vi "Field.vi"(4 "channel 2":T8, 6 "Draw Targets?":T7, 7 "AutoScale":bool=TRUE, 8 "channel for IA State":T9, 10 "Scale mm/pixel":dbl=1.0 format="%#_13g", 11 "channel":T1) -> (2 "Scale Out":dbl, 3 "2D Picture":picture, 5 "AutoScale Out":bool=TRUE)   [LabVIEW 2017]
uses:
  <extravilib>/ChannelInstances/Lossy Stream-t'AI Input.ctl'/)Channel.ctl
  Core/AI Input.ctl
  Core/AI Robot.ctl
  Intel/Functions Enum.ctl
  Intel/AttackerStates.ctl
  Path Planning/RRT/PathDests.ctl
  Path Planning/RRT/PathDest.ctl
  Core/AI Ball.ctl
  Core/Field Size.ctl
  Core/AI Judge.ctl
  Intel/Command Enum.ctl
  Util/Events/Events.ctl
  <extravilib>/ChannelInstances/Lossy Stream-a[.](i32)/)Channel.ctl
  DrawTargets.ctl
  SSL/SSL Field State.ctl
  SSL Detection Frame.ctl
  SSL Detection Robot.ctl
  <vilib>/Analysis/Matrix/Datatypes/RealMatrix.ctl
  SSL Detection Ball.ctl
  <extravilib>/ChannelInstances/Lossy Stream-t'VSS Field State.ctl'/)Channel.ctl
  SSL/VSS Field State.ctl
  <vilib>/Utility/miscctls.llb/LVBoundsTypeDef.ctl
  <extravilib>/ChannelInstances/Lossy Stream-t'VSS Field State.ctl'/Read With Abort.vi
  <extravilib>/ChannelInstances/Lossy Stream-a[.](i32)/Read With Abort.vi
  <extravilib>/ChannelInstances/Lossy Stream-t'AI Input.ctl'/Read With Abort.vi
  <extravilib>/ChannelInstances/Lossy Stream-t'VSS Field State.ctl'/EndpointRead.vi
  <extravilib>/ChannelInstances/Lossy Stream-a[.](i32)/EndpointRead.vi
  <extravilib>/ChannelInstances/Lossy Stream-t'AI Input.ctl'/EndpointRead.vi
  <extravilib>/ChannelInstances/Lossy Stream-t'AI Input.ctl'/)Channel.vi
  <resource>/ChannelSupport/_ChannelSupport/WaitIfNeeded.vi
  <extravilib>/ChannelInstances/Lossy Stream-a[.](i32)/)Channel.vi
  <extravilib>/ChannelInstances/Lossy Stream-t'VSS Field State.ctl'/)Channel.vi
  <extravilib>/ChannelInstances/Lossy Stream-t'AI Input.ctl'.lvlib
  <extravilib>/ChannelInstances/Lossy Stream-a[.](i32).lvlib
  <extravilib>/ChannelInstances/Lossy Stream-t'VSS Field State.ctl'.lvlib
  <vilib>/Analysis/Matrix/NI_Matrix.lvlib
panel:
  in  "element":T2 {"Detection Frame Out"."robots_blue"."height" format="%+4.3f"; "Detection Frame Out"."robots_blue"."pixel_y" format="%+4.3f"; "Detection Frame Out"."robots_blue"."pixel_x" format="%+4.3f"; "Detection Frame Out"."robots_blue"."orientation" format="%+4.3f"; "Detection Frame Out"."robots_blue"."y" format="%+4.3f"; "Detection Frame Out"."robots_blue"."confidence" format="%4.3f"; "Detection Frame Out"."robots_blue"."x" format="%+4.3f"; "Detection Frame Out"."robots_yellow"."height" format="%+4.3f"; "Detection Frame Out"."robots_yellow"."pixel_y" format="%+4.3f"; "Detection Frame Out"."robots_yellow"."pixel_x" format="%+4.3f"; "Detection Frame Out"."robots_yellow"."orientation" format="%+4.3f"; "Detection Frame Out"."robots_yellow"."y" format="%+4.3f"; "Detection Frame Out"."robots_yellow"."confidence" format="%4.3f"; "Detection Frame Out"."robots_yellow"."x" format="%+4.3f"}
  in  "Draw Number":bool=TRUE
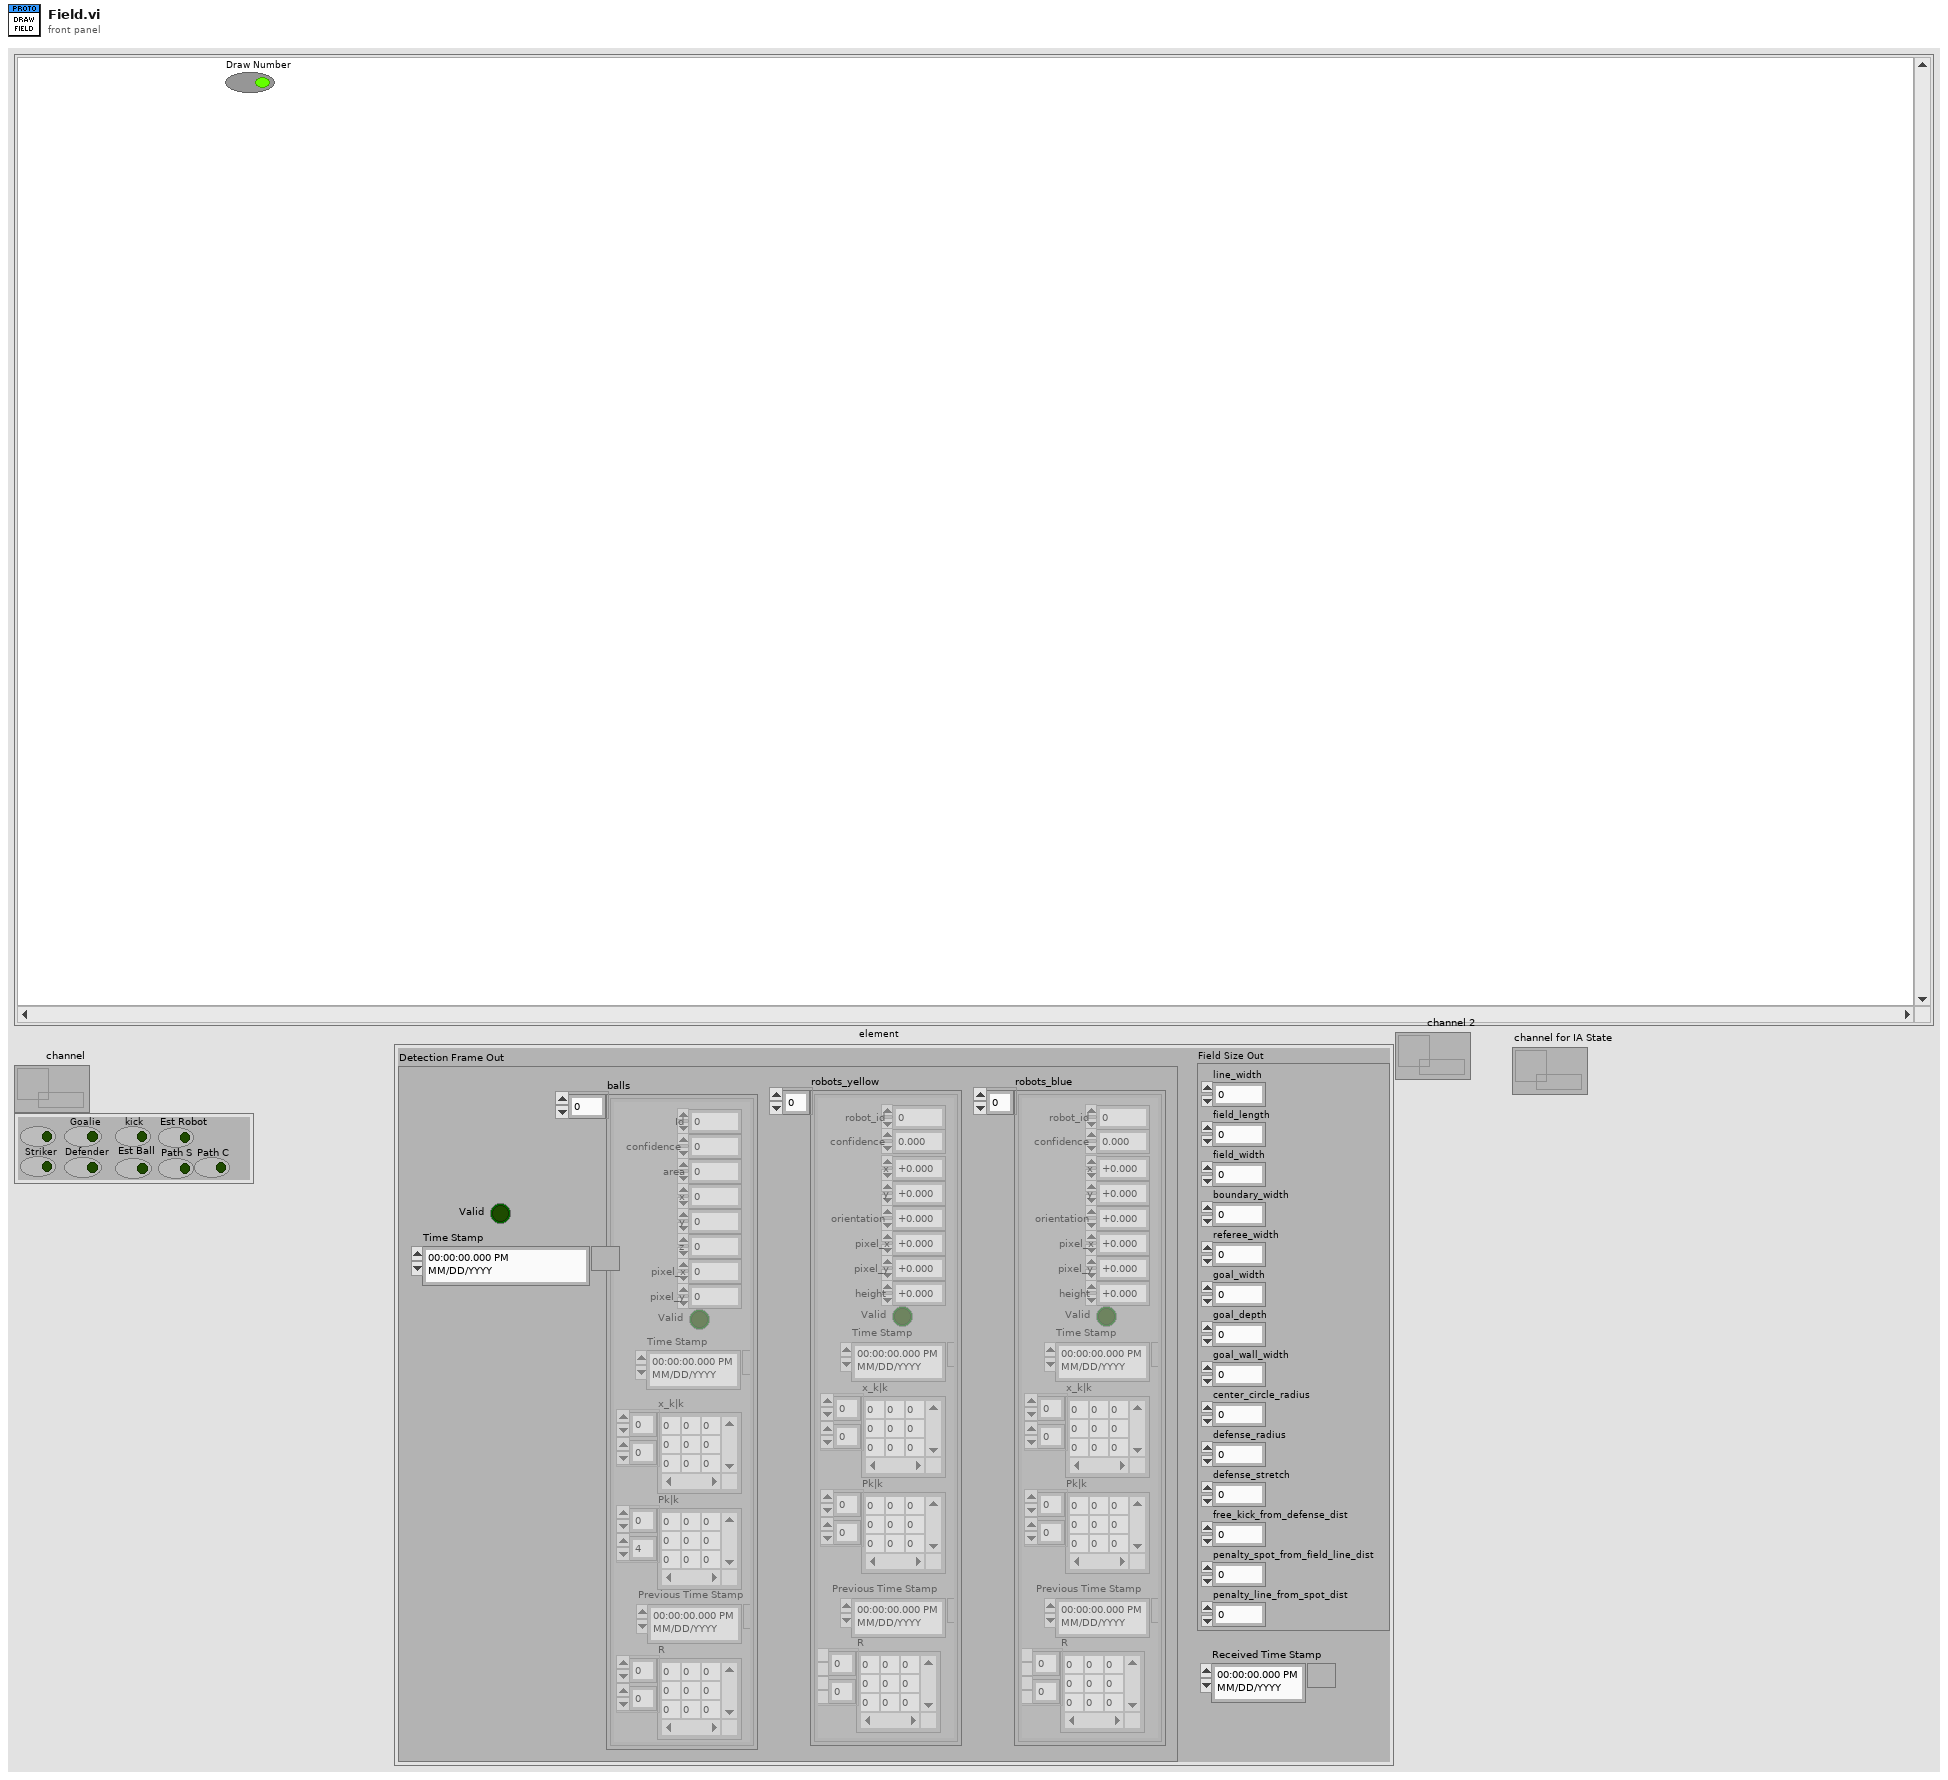
[diagram p1: front panel]
types:
  T1 = typedef "Lossy Stream-t'VSS Field State.ctl'.lvlib/)Channel.ctl" = refnum<queue>
  T2 = typedef "SSL Field State.ctl" = cluster{"Detection Frame Out":T3, "Field Size Out":cluster{"line_width":u32, "field_length":u32, "field_width":u32, "boundary_width":u32, "referee_width":u32, "goal_width":u32, "goal_depth":u32, "goal_wall_width":u32, "center_circle_radius":u32, "defense_radius":u32, "defense_stretch":u32, "free_kick_from_defense_dist":u32, "penalty_spot_from_field_line_dist":u32, "penalty_line_from_spot_dist":u32}, "Received Time Stamp":timestamp}
  T3 = typedef "SSL Detection Frame.ctl" = cluster{"robots_yellow":T4[], "robots_blue":T4[], "balls":T6[], "Valid":bool, "Time Stamp":timestamp}
  T4 = typedef "SSL Detection Robot.ctl" = cluster{"x":sgl, "robot_id":u32, "confidence":sgl, "y":sgl, "orientation":sgl, "pixel_x":sgl, "pixel_y":sgl, "height":sgl, "Valid":bool, "Time Stamp":timestamp, "x_k|k":T5, "Pk|k":T5, "Previous Time Stamp":timestamp, "R":T5}
  T5 = typedef "NI_Matrix.lvlib/RealMatrix.ctl" = dbl[][]
  T6 = typedef "SSL Detection Ball.ctl" = cluster{"x":sgl, "area":u32, "confidence":sgl, "y":sgl, "z":sgl, "pixel_x":sgl, "pixel_y":sgl, "Valid":bool, "Time Stamp":timestamp, "x_k|k":T5, "Pk|k":T5, "Id":u32, "Previous Time Stamp":timestamp, "R":T5}
  T7 = typedef "DrawTargets.ctl" = cluster{"Attacker":bool, "Striker":bool, "Goalie":bool, "Defender":bool, "kick":bool, "Est Ball":bool, "Est Robot":bool, "Path S":bool, "Path C":bool}
  T8 = typedef "Lossy Stream-a[.](i32).lvlib/)Channel.ctl" = refnum<queue>
  T9 = typedef "Lossy Stream-t'AI Input.ctl'.lvlib/)Channel.ctl" = refnum<queue>
  T10 = typedef "LVBoundsTypeDef.ctl" = cluster{"Width":u32, "Height":u32}
  T11 = typedef "VSS Field State.ctl" = cluster{"Detection Frame Out":T3, "Received Time Stamp":timestamp, "Field Size in":cluster{"field_length":u32, "field_width":u32, "goal_width":u32, "goal_depth":u32, "center_circle_radius":u32, "defense_width":u32, "defense_depth":u32, "free_kick_from_defense_dist":u32, "penalty_spot_from_field_line_dist":u32, "penalty_line_from_spot_dist":u32, "half_moon_depth":u32, "half_moon_width":u32}}
  T12 = typedef "AI Input.ctl" = cluster{"our_robots":T13[], "enemy_robots":T13[], "balls":T18[], "geometry":T19, "IA Judge":T20, "Received Timestamp":timestamp, "Events":T22}
  T13 = typedef "AI Robot.ctl" = cluster{"id":u32, "function":T14, "x":dbl, "y":dbl, "orientation":dbl, "v_tangent":dbl, "v_normal":dbl, "v_ang":dbl, "kick_x":dbl, "kick_z":dbl, "dribble":bool, "Timestamp":timestamp, "estimatives":cluster{"est_v_tangent":dbl, "est_v_normal":dbl, "est_vx":dbl, "est_vy":dbl, "Pos Robot Est":dbl[]}, "dest_x_kick":dbl, "dest_y_kick":dbl, "Gap Coord":dbl[], "States":T15, "Path ":dbl[][], "Path  Smooth":dbl[][], "Dest":T16}
  T14 = typedef "Functions Enum.ctl" = enum16{"Attacker", "Goalie", "Defender", "Striker", "Goto 0", "Dummy", "Kicker", "ZigZag"}
  T15 = typedef "AttackerStates.ctl" = enum16{"Pass", "GoToTangent", "BallGetting", "GoToKick", ""}
  T16 = typedef "PathDests.ctl" = T17[]
  T17 = typedef "PathDest.ctl" = cluster{"dest_x":dbl, "dest_y":dbl, "dest_orientation":dbl, "dest_vel":dbl}
  T18 = typedef "AI Ball.ctl" = cluster{"x":dbl, "y":dbl, "timestamp":timestamp, "Vel_x":dbl, "Vel_y":dbl, "Pos Bola Est":dbl[]}
  T19 = typedef "Field Size.ctl" = cluster{"line_width":u32, "field_length":u32, "field_width":u32, "boundary_width":u32, "referee_width":u32, "goal_width":u32, "goal_depth":u32, "goal_wall_width":u32, "center_circle_radius":u32, "defense_radius":u32, "defense_stretch":u32, "free_kick_from_defense_dist":u32, "penalty_spot_from_field_line_dist":u32, "penalty_line_from_spot_dist":u32}
  T20 = typedef "AI Judge.ctl" = cluster{"stage":string, "command":string, "our_goalie_id":dbl, "enemy_goalie_id":dbl, "command enum":T21, "Time":enum16{"Azul", "Amarelo"}}
  T21 = typedef "Command Enum.ctl" = enum16{"Halt", "Stop", "Force Start", "PKA Normal Start", "Prepare Kickoff Ally", "PKE Normal Start", "Prepare Kickoff Enemy", "Prepare Penalty Ally", "PPA Normal Start", "Prepare Penalty Enemy", "PPE Normal Start", "Direct Free Enemy", "Direct Free Ally", "Indirect Free Enemy", "Indirect Free Ally", "Timeout Enemy", "Timeout Ally", "Goal Enemy", "Goal Ally", "Ball Placement Enemy", "Ball Placement Ally", "Normal Half Time", "Extra Time Break", "Extra Half Time", "None", "Post Game"}
  T22 = typedef "Events.ctl" = cluster{"Touch":bool, "Ball out":bool, "id touch":dbl, "Ball out of \nVision":bool, "Ball inside \nGoalie area":bool, "Robot not responding":bool, "Robots responding status":dbl[], "Enemy Ball \nPossession":bool, "Pass State":bool, "id end of pass":dbl, "Kick":bool, "Id ini Possession":dbl, "Ball Possesion":bool, "Id Possesion":dbl}
  T23 = cluster{"field_length":u32, "field_width":u32, "goal_width":u32, "goal_depth":u32, "center_circle_radius":u32, "defense_width":u32, "defense_depth":u32, "free_kick_from_defense_dist":u32, "penalty_spot_from_field_line_dist":u32, "penalty_line_from_spot_dist":u32, "half_moon_depth":u32, "half_moon_width":u32}
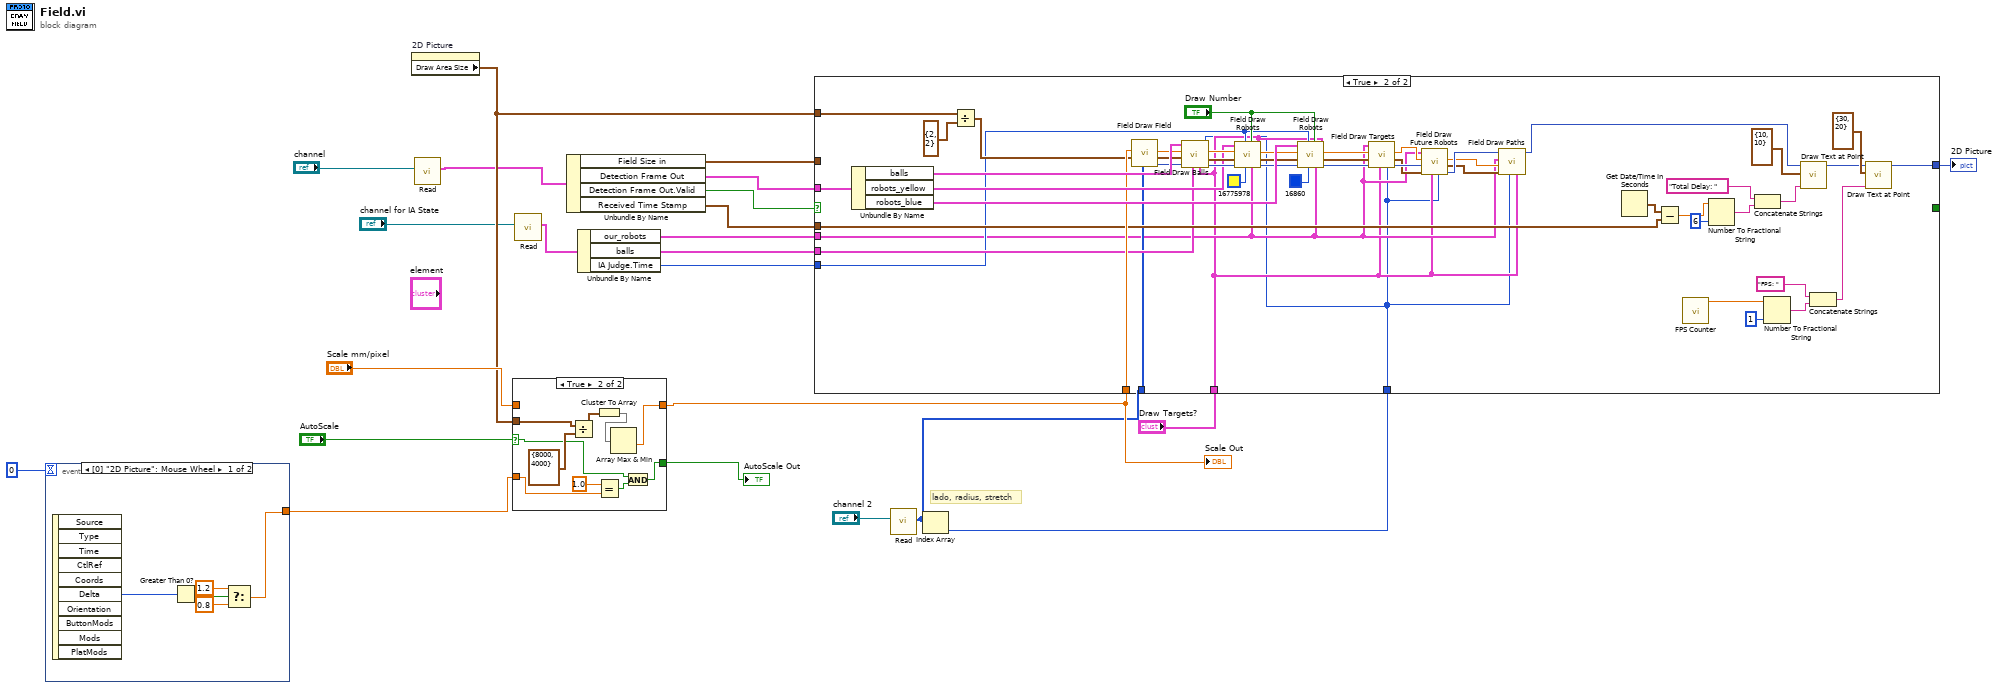
[diagram p0: block diagram]
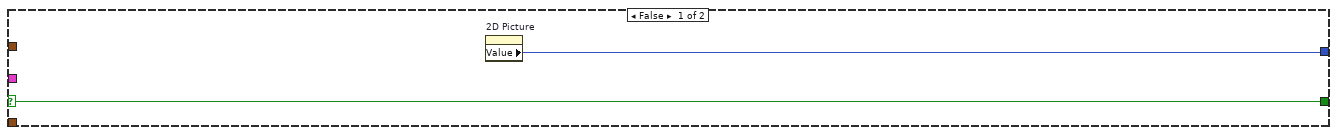
[diagram p2: hidden frame]
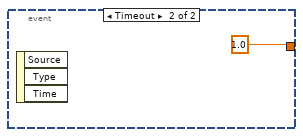
[diagram p3: hidden frame]
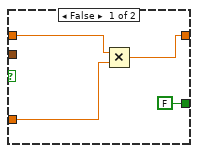
[diagram p4: hidden frame]
diagram:
  # "lado, radius, stretch"
  n1 = event shown="[0] \"2D Picture\": Mouse Wheel" {
    selector: _ -> [_ _]
    dyn-events: _ -> [_ _]
    timeout: 0 -> [_ _]
    tunnel: [w24 1.0] -> w21
    event "2D Picture": Mouse Wheel {
      n2 = event-data() -> ("Delta"=w28:i32)  [unwired: 1 in, 9 out]
      n3 = Greater Than 0?(x=w28) -> (x > 0?=w27:bool)
      n4 = Select(t=1.2, s=w27, f=0.8) -> (s? t:f=w24:dbl)
    }
    event Timeout {
      n5 = event-data() -> ()  [unwired: 1 in, 3 out]
    }
  }
  n6 = property on="2D Picture" class="Pict"() -> ("Draw Area Size"=w20:T10)  [unwired: 2 in, 2 out]
  n7 = call <extravilib>:"Read.vi"("channel"="channel") -> ("element"=w1:T11)  [unwired: 5 in, 5 out]
  n8 = case shown="True" "AutoScale" {
    selector: "AutoScale" -> [_ w35]
    tunnel: "Scale mm/pixel" -> [w33 _]
    tunnel: [w32 w39] -> w15
    tunnel: w20 -> [_ w43]
    tunnel: w21 -> [w31 w38]
    tunnel: [FALSE w36] -> w18
    frame False {
      n9 = Multiply(x=w33, y=w31) -> (x*y=w32:dbl)
    }
    frame True {
      n10 = Divide(x=w43, y=T10 {"Width"=8000, "Height"=4000}) -> (x/y=w41:cluster{"Width":dbl, "Height":dbl})
      n11 = Cluster To Array(cluster=w41) -> (array=w40:dbl[])
      n12 = Equal?(x=1.0, y=w38) -> (x = y?=w34:bool)
      n13 = Array Max & Min(array=w40) -> (min value=w39:dbl)  [unwired: 3 out]
      n14 = And(x=w35, y=w34) -> (x .and. y?=w36:bool)
    }
  }
  "Scale Out" <- w15
  "AutoScale Out" <- w18
  n15 = call <extravilib>:"Read.vi"("channel"="channel for IA State") -> ("element"=w12:T12)  [unwired: 5 in, 5 out]
  n16 = Unbundle By Name(w1) -> ("Field Size in"=w16:T23, "Detection Frame Out"=w17:T3, "Detection Frame Out.Valid"=w14:bool, "Received Time Stamp"=w13:timestamp)
  n17 = Unbundle By Name(w12) -> ("our_robots"=w3:T13[], "balls"=w7:T18[], "IA Judge.Time"=w4:enum16{"Azul", "Amarelo"})
  n18 = call <extravilib>:"Read.vi"("channel"="channel 2") -> ("element"=w5:i32[])  [unwired: 5 in, 5 out]
  n19 = Index Array(array=w5) -> (element=w10:i32)  [unwired: 1 in]
  n20 = case shown="True" w14 {
    selector: w14 -> [w45 _]
    tunnel: w20 -> [_ w96]
    tunnel: [w44 w70] -> w9
    tunnel: w17 -> [_ w84]
    tunnel: w16 -> [_ _]
    tunnel: w15 -> [_ w83]
    tunnel: [w45 _] -> _
    tunnel: w13 -> [_ w77]
    tunnel: w3 -> [_ w49]
    tunnel: "Draw Targets?" -> [_ w48]
    tunnel: w10 -> [_ w46]
    tunnel: w7 -> [_ w60]
    tunnel: w5 -> [_ w54]
    tunnel: w4 -> [_ w53]
    frame False {
      n21 = property on="2D Picture" class="Pict"() -> ("Value"=w44:picture)  [unwired: 2 in, 2 out]
    }
    frame True {
      n22 = Unbundle By Name(w84) -> ("balls"=w95:T6[], "robots_yellow"=w91:T4[], "robots_blue"=w90:T4[])
      n23 = Divide(x=w96, y=T10 {"Width"=2, "Height"=2}) -> (x/y=w80:cluster{"Width":dbl, "Height":dbl})
      n24 = call "Field Draw Field.vi"("Lado,radius, stretch"=w54, "Offset"=w80, "Scale"=w83) -> ("new picture out"=w81:picture, "Offset Out"=w79:cluster{"Width":dbl, "Height":dbl}, "Scale Out"=w82:dbl)  [unwired: 6 in]
      n25 = call "Field Draw Balls.vi"("Lado"=w46, "Draw Targets?"=w48, "balls"=w60, "Picture In"=w81, "Offset"=w79, "Scale"=w82, "Balls"=w95) -> ("Picture Out"=w94:picture, "Offset Out"=w93:cluster{"Width":dbl, "Height":dbl}, "Scale Out"=w92:dbl)  [unwired: 2 in]
      n26 = call "Field Draw Robots.vi"("Draw Targets?"=w48, "our_robots"=w49, "Draw Number"="Draw Number", "color(black)"=u32 16775978, "IA Judge.Time"=w53, "Picture In"=w94, "Offset"=w93, "Scale"=w92, "Detection Robots"=w91) -> ("Picture Out"=w87:picture, "Offset Out"=w88:cluster{"Width":dbl, "Height":dbl}, "Scale Out"=w89:dbl)
      n27 = call "Field Draw Robots.vi"("Draw Targets?"=w48, "our_robots"=w49, "Draw Number"="Draw Number", "color(black)"=u32 16860, "IA Judge.Time"=w53, "Picture In"=w87, "Offset"=w88, "Scale"=w89, "Detection Robots"=w90) -> ("Picture Out"=w62:picture, "Offset Out"=w61:cluster{"Width":dbl, "Height":dbl}, "Scale Out"=w59:dbl)
      n28 = call "Field Draw Targets.vi"("Lado"=w46, "Draw Targets?"=w48, "Picture In"=w62, "Offset"=w61, "Scale"=w59, "our_robots"=w49) -> ("Picture Out"=w58:picture, "Offset Out"=w57:cluster{"Width":dbl, "Height":dbl}, "Scale Out"=w56:dbl)  [unwired: 3 in]
      n29 = call "Field Draw Future Robots.vi"("Lado"=w46, "Draw Targets?"=w48, "Offset"=w57, "Picture In"=w58, "Scale"=w56, "our_robots"=w49) -> ("Picture Out"=w52:picture, "Offset Out"=w50:cluster{"Width":dbl, "Height":dbl}, "Scale Out"=w51:dbl)  [unwired: 3 in]
      n30 = call "Field Draw Paths.vi"("Draw Targets?"=w48, "Lado"=w46, "Offset"=w50, "Scale mm/pixel"=w51, "our_robots"=w49, "picture in"=w52) -> ("picture out"=w47:picture)  [unwired: 5 in]
      n31 = Get Date/Time In Seconds() -> (seconds since 1Jan1904=w76:timestamp)
      n32 = Subtract(x=w76, y=w77) -> (x-y=w75:dbl)
      n33 = call "FPS Counter.vi"() -> ("Numeric"=w66:dbl)  [unwired: 11 in]
      n34 = Number To Fractional String(number=w75, precision (6)=i16 6) -> (F-format string=w73:string)  [unwired: 2 in]
      n35 = Concatenate Strings("Total Delay: " ("text"), w73) -> (w72:string)
      n36 = Number To Fractional String(number=w66, precision (6)=i16 1) -> (F-format string=w68:string)  [unwired: 2 in]
      n37 = call <vilib>:"Draw Text at Point.vi"("text"=w72, "origin"=cluster{"x":i16, "y":i16} {"x"=10, "y"=10}, "picture"=w47) -> ("new picture"=w55:picture)  [unwired: 7 in, 1 out]
      n38 = Concatenate Strings("FPS: " ("text"), w68) -> (w64:string)
      n39 = call <vilib>:"Draw Text at Point.vi"("text"=w64, "origin"=cluster{"x":i16, "y":i16} {"x"=30, "y"=20}, "picture"=w55) -> ("new picture"=w70:picture)  [unwired: 7 in, 1 out]
    }
  }
  "2D Picture" <- w9
